vi "数据显示.vi"() -> ()   [LabVIEW 2016]
panel:
  in  "数组":string[][](array[string])
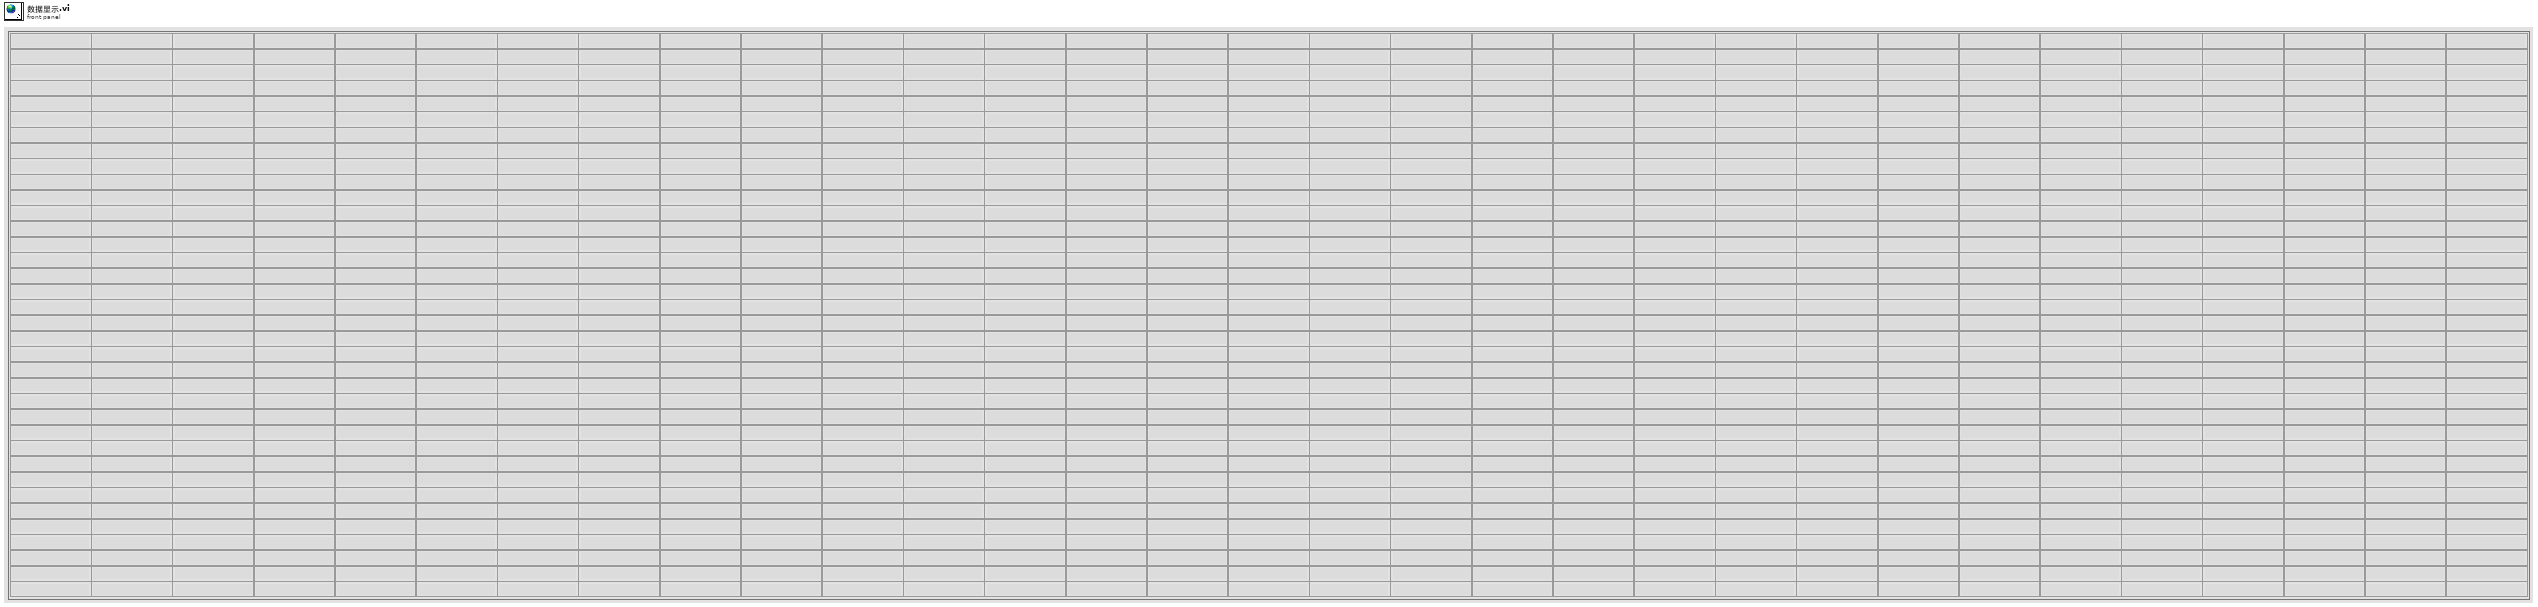
[diagram p1: front panel]
diagram:
